vi "Populate Tree.vi"(5 "Pre-Clear Tree?(T)":bool=TRUE, 7 "Close Reference?(T)":bool=TRUE, 8 "error in (no error)":errorcluster, 10 "Hierarchy Filter(empty=all)":string, 11 "TreeControl in":refnum<vi>) -> (0 "error out":errorcluster, 1 "Success?":bool, 3 "Classes found":string[](array[string]))   [LabVIEW 2020, in "ClassLoader.lvlib"]
doc: "Populate a tree control with a the hierarchy loaded using the given Hierarchy Filter."
uses:
  ClassLoader.lvlib
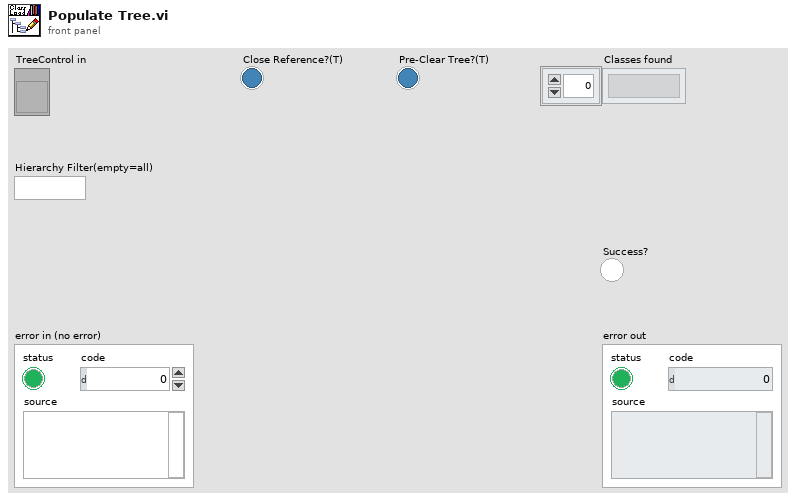
[diagram p1: front panel]
types:
  T1 = cluster{"Left Cell String":string, "Child Text":string[], "Child Tag":string, "Item Indent":i32, "Child Only?":bool, "Glyph Index":i32}
  T2 = typedef "ClassLoader.lvlib/Ctl_Hierarchy Cluster.ctl" = cluster{"Hierarchy":string[]}
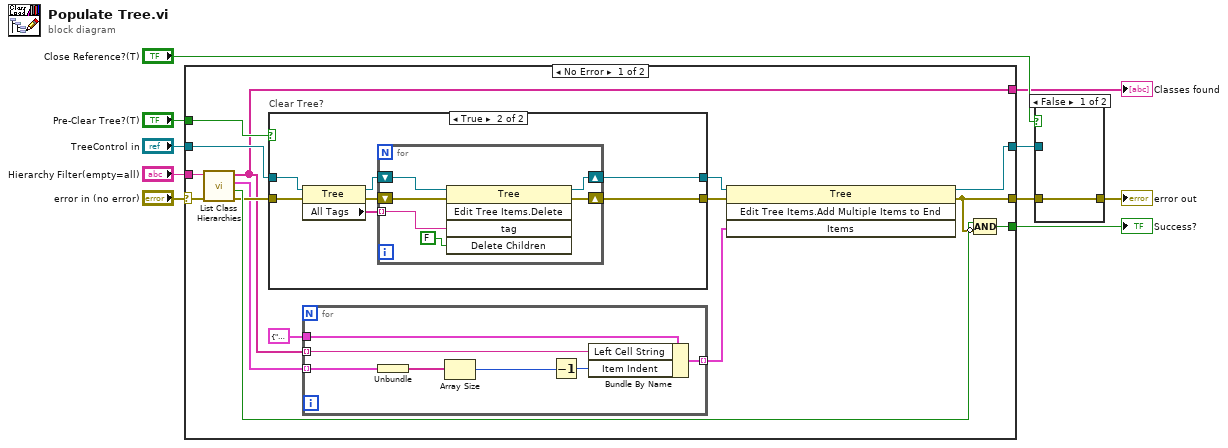
[diagram p0: block diagram]
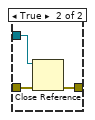
[diagram p4: hidden frame]
diagram:
  n1 = case shown="No Error" "error in (no error)" {
    selector: "error in (no error)" -> [w12 w49]
    tunnel: [w25 _] -> w10
    tunnel: "Pre-Clear Tree?(T)" -> [w23 _]
    tunnel: "TreeControl in" -> [w21 w48]
    tunnel: [w17 w48] -> w5
    tunnel: [w16 _] -> w4
    tunnel: "Hierarchy Filter(empty=all)" -> [w13 _]
    tunnel: [w11 w49] -> w1
    frame No Error {
      n2 = call "List Class Hierarchies.vi"("error in (no error)"=w12, "Hierarchy Filter(empty=all)"=w13) -> ("error out"=w22:errorcluster, "Success?"=w24:bool, "Class Hierarchies"=w15:T2[], "Classes found"=w16:string[])  [unwired: 6 in]
      n3 = case "Clear Tree?" shown="True" w23 {
        tunnel: [w27 w34] -> w19
        tunnel: [w26 w33] -> w20
        tunnel: w21 -> [w27 w32]
        tunnel: w22 -> [w26 w31]
        frame False {
        }
        frame True {
          n4 = property class="Tree"(reference=w32, error in=w31) -> (reference out=w29:refnum<vi>, error out=w30:errorcluster, "All Tags"=w28:string[])
          n5 = for {
            shift-right: [w38] -> w33
            shift-left: w30 -> [w39]
            shift-right: [w40] -> w34
            shift-left: w29 -> [w37]
            tunnel: w28 -> [w35] mode=indexing
            n6 = invoke class="Tree" method="Edit Tree Items.Delete"(reference=w37, error in=w39, "tag"=w35, "Delete Children"=FALSE) -> (reference out=w40:refnum<vi>, error out=w38:errorcluster)  [unwired: 1 in, 3 out]
          }
        }
      }
      n7 = for {
        tunnel: T1 {"Left Cell String"="", "Child Text"=[], "Child Tag"="", "Item Indent"=0, "Child Only?"=FALSE, "Glyph Index"=0} ("Item") -> [w47]
        tunnel: w15 -> [w46] mode=indexing
        tunnel: w16 -> [w43] mode=indexing
        tunnel: [w41] -> w18 mode=indexing
        n8 = Unbundle(w46) -> ("Hierarchy"=w45:string[])
        n9 = Array Size(array=w45) -> (size(s)=w44:i32)
        n10 = Decrement(x=w44) -> (x-1=w42:i32)
        n11 = Bundle By Name(cluster=w47, "Left Cell String"=w43, "Item Indent"=w42) -> (w41:T1)
      }
      n12 = invoke class="Tree" method="Edit Tree Items.Add Multiple Items to End"(reference=w19, error in=w20, "Items"=w18) -> (reference out=w17:refnum<vi>, error out=w11:errorcluster)  [unwired: 1 in, 2 out]
      n13 = Compound Arithmetic op=AND(w24, invert w11) -> (w25:bool)
    }
    frame Error {
    }
  }
  "Success?" <- w10
  "Classes found" <- w4
  n14 = case shown="False" "Close Reference?(T)" {
    tunnel: w1 -> [w50 w53]
    tunnel: w5 -> [_ w52]
    tunnel: [w50 w51] -> w9
    frame False {
    }
    frame True {
      n15 = Close Reference(reference=w52, error in (no error)=w53) -> (error out=w51:errorcluster)
    }
  }
  "error out" <- w9
